vi "Write Path to DLL.vi"(8 "error in (no error)":errorcluster, 10 "Path to DLL":path, 11 "PC in":refnum<class "PC.lvclass">) -> (0 "error out":errorcluster, 3 "PC out":refnum<class "PC.lvclass">)   [LabVIEW 2017, in "PC.lvclass"]
uses:
  PC.lvclass
  PC.lvclass/PC.ctl
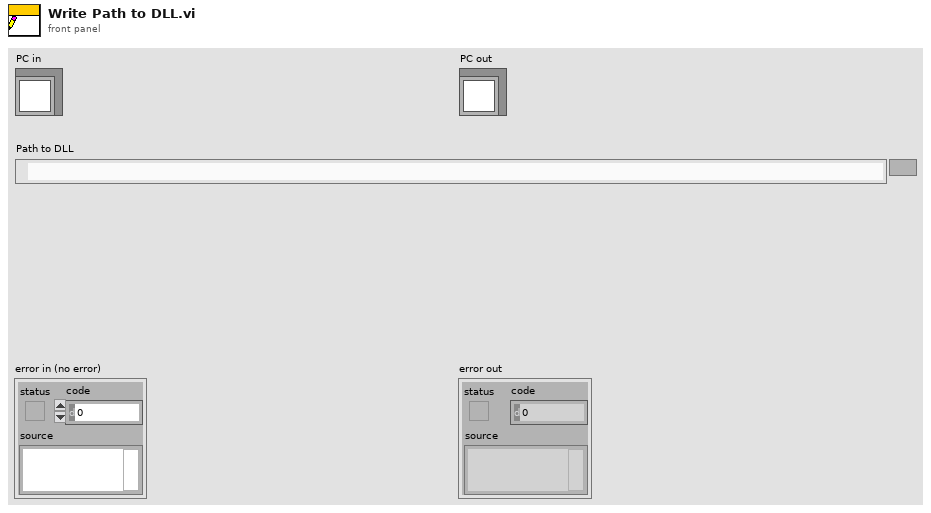
[diagram p1: front panel]
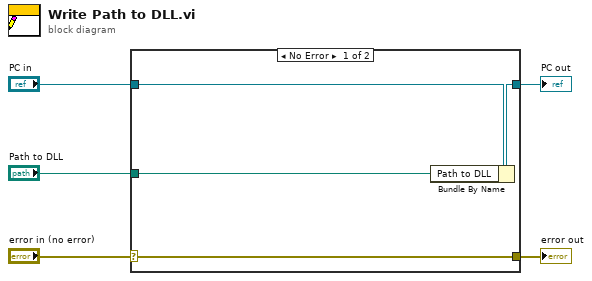
[diagram p0: block diagram]
diagram:
  n1 = case shown="No Error" "error in (no error)" {
    selector: "error in (no error)" -> [w9 w10]
    tunnel: [w9 w10] -> w4
    tunnel: [w7 w11] -> w2
    tunnel: "PC in" -> [w8 w11]
    tunnel: "Path to DLL" -> [w6 _]
    frame No Error {
      n2 = Bundle By Name(cluster=w8, "Path to DLL"=w6) -> (w7:refnum<class "PC.lvclass">)
    }
    frame Error {
    }
  }
  "error out" <- w4
  "PC out" <- w2
